vi "logSummaryState.vi"(8 "error in (no error)":errorcluster, 10 "EventSummaryState":T1, 11 "M1M3SAL in":refnum<class "M1M3SAL.lvclass">) -> (0 "error out":errorcluster, 3 "M1M3SAL out":refnum<class "M1M3SAL.lvclass">)   [LabVIEW 2016, in "M1M3SupportCommunicator.lvlib" / "M1M3SAL.lvclass"]
uses:
  M1M3SAL.lvclass
  DataTypes/Topics/EventSummaryState.ctl
  DataTypes/Topics/Parts/Timestamp.ctl
  DataTypes/Topics/Parts/SummaryStates.ctl
  DataTypes/MessageHeader.ctl
  DataTypes/MessageTypes.ctl
  DataTypes/MessageTopics.ctl
  Common_RT_Utilities/U8ArrayBuilderAutoIndexing/U8ArrayBuilderAutoIndexing.lvclass
  M1M3SupportCommunicator.lvlib
  DataTypes/Topics/M1M3SupportTopics.lvlib
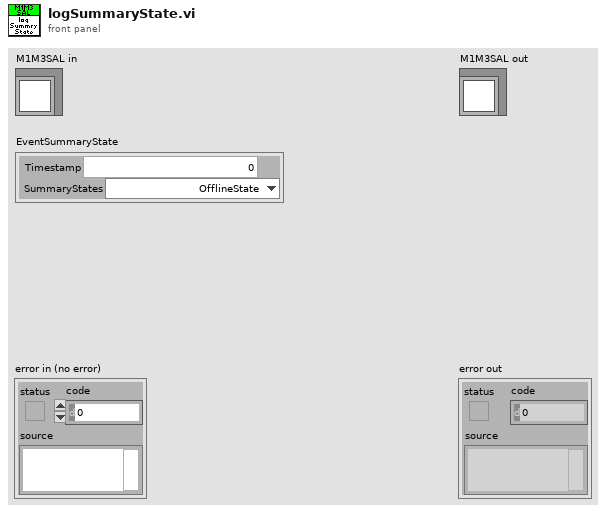
[diagram p1: front panel]
types:
  T1 = typedef "M1M3SupportTopics.lvlib/EventSummaryState.ctl" = cluster{"Timestamp":T2, "SummaryStates":T3}
  T2 = typedef "M1M3SupportTopics.lvlib/Timestamp.ctl" = dbl
  T3 = typedef "M1M3SupportTopics.lvlib/SummaryStates.ctl" = enum16{"OfflineState", "StandbyState", "DisabledState", "EnabledState", "FaultState"}
  T4 = typedef "M1M3SupportCommunicator.lvlib/MessageHeader.ctl" = cluster{"Type":T5, "Topic":T6, "Size":i32}
  T5 = typedef "M1M3SupportCommunicator.lvlib/MessageTypes.ctl" = enum8{"None", "PutSample", "GetNextSample", "LogEvent", "GetEvent", "IssueCommand", "CommandId", "WaitForCompletion", "AcceptCommand", "AckCommand"}
  T6 = typedef "M1M3SupportCommunicator.lvlib/MessageTopics.ctl" = enum8{"None", "ForceActuatorData", "MirrorForceData", "HardpointData", "AirData", "DynamicData", "FPGAData", "IMSData", "ForceActuatorStatus", "ElevationData", "HardpointStatus", "HardpointActuatorChase", "AirStatus", "ForceActuatorSafetyChecks", "ForceActuatorTest", "ActuatorBroadcastCounter", "StatusChecks", "CellChecks", "HardpointActuatorBreakaway", "RaiseMirrorComplete", "ILCCommunication", "ElevationAngleChecks", "DetailedState", "ServoLoops", "ForceActuatorInfo", "LowerMirrorComplete", "HardpointActuatorInfo", "SettingsApplied", "ErrorCode", "StartupChecks", "SummaryState", "SettingVersions", "ActuatorTestStatus", "AppliedSettingsMatchStart", "Enable", "EnterMaintenance", "Standby", "AbortLowerM1M3", "ApplyAberrationByForces", "ApplyAOSCorrectionByBendingModes", "ClearAOSCorrection", "Start", "RaiseM1M3", "TestForceActuator", "LowerM1M3", "ApplyAOSCorrectionByForces", "Disable", "ApplyAberationByBendingMode", "TestHardpoint", "ManipulateM1M3", "ClearAberration", "Exit", "TestAir", "AbortRaiseM1M3", "MoveHardpointActuators", "ExitMaintenance", "Shutdown"}
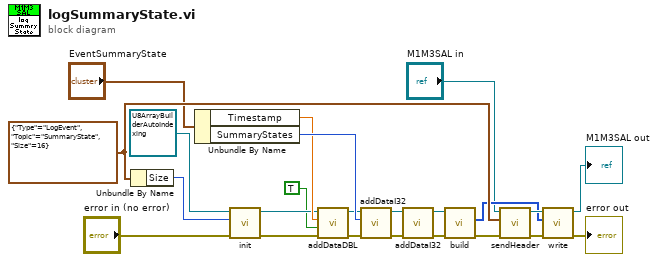
[diagram p0: block diagram]
diagram:
  w22 = T4 {"Type"=enum."LogEvent", "Topic"=enum."SummaryState", "Size"=16} ("MessageHeader")
  n1 = Unbundle By Name(w22) -> ("Size"=w21:i32)
  n2 = Unbundle By Name("EventSummaryState") -> ("Timestamp"=w10:T2, "SummaryStates"=w11:T3)
  n3 = call "init.vi"("error in (no error)"="error in (no error)", "Size"=w21, "U8ArrayBuilderAutoIndexing in"=refnum<class "U8ArrayBuilderAutoIndexing.lvclass"> refnum ("RTUtilities.lvlib:U8ArrayBuilderAutoIndexing.lvclass")) -> ("error out"=w5:errorcluster, "U8ArrayBuilderAutoIndexing out"=w9:refnum<class "U8ArrayBuilderAutoIndexing.lvclass">)  [unwired: 7 in]
  n4 = call "addDataDBL.vi"("error in (no error)"=w5, "OverrideSwapBytes"=TRUE, "Data"=w10, "U8ArrayBuilderAutoIndexing in"=w9) -> ("error out"=w7:errorcluster, "U8ArrayBuilderAutoIndexing out"=w8:refnum<class "U8ArrayBuilderAutoIndexing.lvclass">)  [unwired: 6 in]
  n5 = call "addDataI32.vi"("error in (no error)"=w7, "Data"=w11, "U8ArrayBuilderAutoIndexing in"=w8) -> ("error out"=w3:errorcluster, "U8ArrayBuilderAutoIndexing out"=w4:refnum<class "U8ArrayBuilderAutoIndexing.lvclass">)  [unwired: 7 in]
  n6 = call "addDataI32.vi"("error in (no error)"=w3, "U8ArrayBuilderAutoIndexing in"=w4) -> ("error out"=w2:errorcluster, "U8ArrayBuilderAutoIndexing out"=w1:refnum<class "U8ArrayBuilderAutoIndexing.lvclass">)  [unwired: 8 in]
  n7 = call "build.vi"("error in (no error)"=w2, "U8ArrayBuilderAutoIndexing in"=w1) -> ("error out"=w17:errorcluster, "Array"=w18:u8[])  [unwired: 7 in, 1 out]
  n8 = call "sendHeader.vi"("error in (no error)"=w17, "MessageHeader"=w22, "M1M3SAL in"="M1M3SAL in") -> ("error out"=w16:errorcluster, "M1M3SAL out"=w19:refnum<class "M1M3SAL.lvclass">)  [unwired: 7 in]
  n9 = call "write.vi"("error in (no error)"=w16, "Data"=w18, "M1M3SAL in"=w19) -> ("error out"=→"error out":errorcluster, "M1M3SAL out"=→"M1M3SAL out":refnum<class "M1M3SAL.lvclass">)  [unwired: 7 in]
